vi "Opgave 6.1 Build_String 15 udgave.vi"(8 "String 2":string="volts DC: +1.26E+1", 9 "Trailer":string="volts", 10 "Numeric":dbl=3.0, 11 "Header":string="the measure is") -> (0 "Offset Past Match":i32=-1, 1 "Number Out":dbl, 2 "String Length":i32=8, 3 "Combined string":string=" 0,0000 ")   [LabVIEW 2015]
panel:
  in  "Return":bool
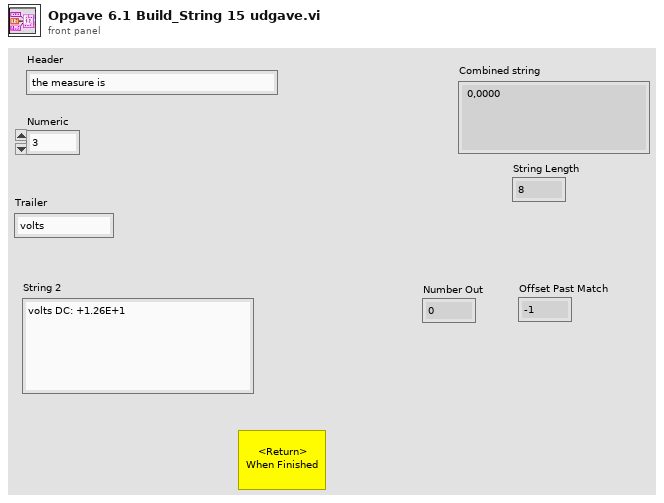
[diagram p1: front panel]
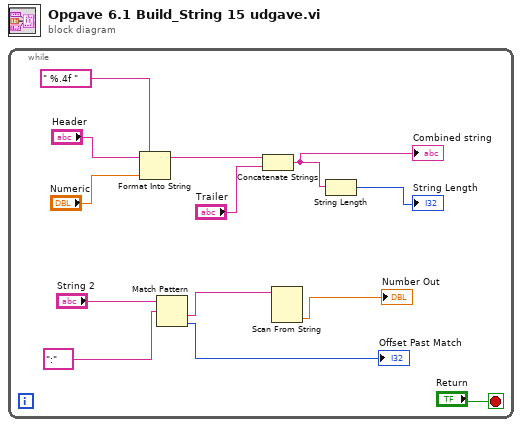
[diagram p0: block diagram]
diagram:
  n1 = while {
    stop <- "Return" stop-if-true
    n2 = Format Into String "Format Into String"(format string=" %.4f ", initial string="Header", "Numeric") -> (resulting string=w9:string)  [unwired: 1 in, 1 out]
    n3 = Match Pattern(string="String 2", regular expression=":") -> (after substring=w4:string, offset past match=→"Offset Past Match":i32)  [unwired: 1 in, 2 out]
    n4 = Concatenate Strings "Concatenate Strings"(w9, "Trailer") -> (w7:string)
    "Combined string" <- w7
    n5 = Scan From String "Scan From String"(input string=w4) -> (output 1=→"Number Out":dbl)  [unwired: 4 in, 3 out]
    n6 = String Length(string=w7) -> (length=→"String Length":i32)
  }
